vi "Advance past Comment.vi"(7 "JSON":string, 9 "Offset":i32) -> (1 "Offset past match":i32, 2 "Line End Comment":bool, 3 "State":T1)   [LabVIEW 2020, in "JSONtext.lvlib"]
uses:
  <vilib>/JDP Science/JSONtext/JSONtext.lvlib
  <vilib>/JDP Science/JSONtext/Parsing/Parsing State.ctl
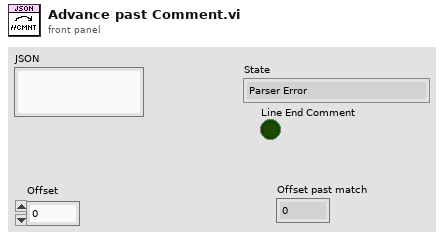
[diagram p1: front panel]
types:
  T1 = typedef "JSONtext.lvlib/Parsing State.ctl" = enum16{"Parser Error", "Object", "Array", "String", "Number/Other", "Leading Whitespace", "Object end", "Array end", "Value end"}
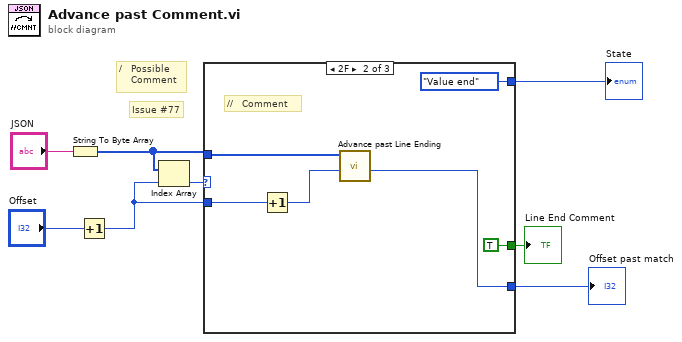
[diagram p0: block diagram]
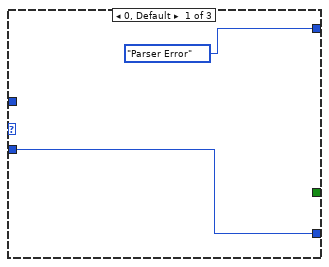
[diagram p2: hidden frame]
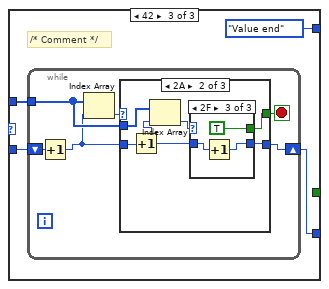
[diagram p3: hidden frame]
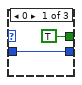
[diagram p5: hidden frame]
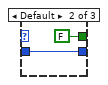
[diagram p6: hidden frame]
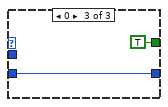
[diagram p7: hidden frame]
diagram:
  # "Issue #77"
  # "/   Possible \n    Comment"
  n1 = String To Byte Array(string="JSON") -> (unsigned byte array=w6:u8[])
  n2 = Increment(x="Offset") -> (x+1=w2:i32)
  n3 = Index Array(array=w6, index=w2) -> (element=w7:u8)
  n4 = case shown="2F" w7 {
    tunnel: w6 -> [_ w16 w20]
    tunnel: w2 -> [w9 w15 w18]
    tunnel: [w9 w14 w19] -> w3
    tunnel: [Parsing_State."Parser Error" ("t") Parsing_State."Value end" ("t") Parsing_State."Value end" ("t")] -> w4
    tunnel: [_ TRUE _] -> w1
    frame 0, Default {
    }
    frame 47 {
      # "//   Comment"
      n5 = Increment(x=w15) -> (x+1=w13:i32)
      n6 = call <vilib>:"Advance past Line Ending.vi"("Offset"=w13, "JSON"=w16) -> ("Offset after Line Ending"=w14:i32)  [unwired: 9 in]
    }
    frame 42 {
      # "/* Comment */"
      n7 = while {
        tunnel: w20 -> [w23]
        shift-right: [w24] -> w19
        shift-left: w18 -> [w22]
        stop <- w25 stop-if-true
        n8 = Increment(x=w22) -> (x+1=w21:i32)
        n9 = Index Array(array=w23, index=w21) -> (element=w26:u8)
        n10 = case shown="2A" w26 {
          tunnel: w21 -> [w27 w31 w42]
          tunnel: [_ w28 TRUE] -> w25
          tunnel: [w27 w29 w42] -> w24
          tunnel: w23 -> [_ w30 _]
          frame Default {
          }
          frame 42 {
            n11 = Increment(x=w31) -> (x+1=w32:i32)
            n12 = Index Array(array=w30, index=w32) -> (element=w33:u8)
            n13 = case shown="2F" w33 {
              tunnel: [TRUE FALSE TRUE] -> w28
              tunnel: w32 -> [w35 w37 w39]
              tunnel: [w35 w37 w38] -> w29
              frame 0 {
              }
              frame Default {
              }
              frame 47 {
                n14 = Increment(x=w39) -> (x+1=w38:i32)
              }
            }
          }
          frame 0 {
          }
        }
      }
    }
  }
  "State" <- w4
  "Offset past match" <- w3
  "Line End Comment" <- w1
